vi "Trap2-Test-05-16.vi"() -> ()   [LabVIEW 2010]
panel:
  in  "stop":bool
  out "UTemp[V]Trap2":fxp<+/-,16,4> format="%.25g"
  in  "Per[us]Trap2":u32 caption="PerTrap2[us]"
  in  "warten[us]Trap2":u32=200
  in  "UTempSPTrap2":fxp<+/-,16,4> format="%.14g"
  in  "UTempMaxTrap2":fxp<+/-,16,4> format="%.14g"
  in  "PIDTrap2":T1 {"proportional gain (Kc)" format="%.11g"; "integral gain (Kc*Ts/Ti)" format="%.11g"; "derivative gain (Kc*Td/Ts)" format="%.11g"}
  in  "Heizen?Trap2":bool
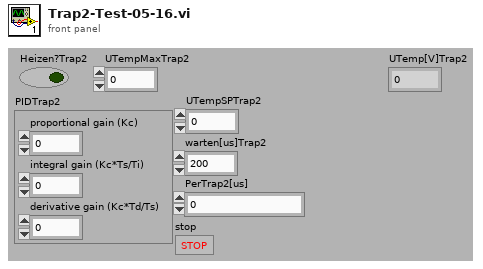
[diagram p1: front panel]
types:
  T1 = cluster{"proportional gain (Kc)":fxp<+/-,16,8>, "integral gain (Kc*Ts/Ti)":fxp<+/-,16,8>, "derivative gain (Kc*Td/Ts)":fxp<+/-,16,8>}
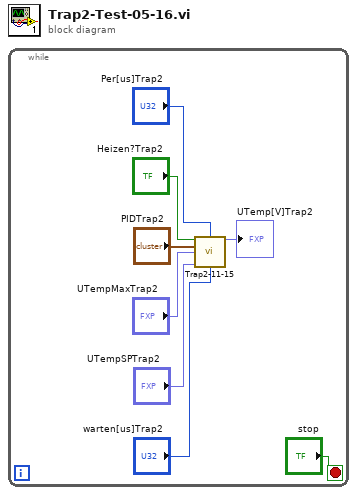
[diagram p0: block diagram]
diagram:
  n1 = while {
    stop <- "stop" stop-if-true
    n2 = call "Trap2-11-15.vi"("Heizen?Trap2"="Heizen?Trap2", "Per[us]Trap2"="Per[us]Trap2", "PIDTrap2"="PIDTrap2", "UTempMaxTrap2"="UTempMaxTrap2", "UTempSPTrap2"="UTempSPTrap2", "warten[us]Trap2"="warten[us]Trap2") -> ("UTemp[V]Trap2"=→"UTemp[V]Trap2":fxp<+/-,16,4>)  [unwired: 9 in]
  }
